vi "Resize Buffer.vi"(8 "error in (no error)":errorcluster, 10 "New Size":i32=-1, 11 "2D U16 DVR Array in":refnum<class "2D U16 DVR Array.lvclass">) -> (0 "error out":errorcluster, 3 "2D U16 DVR Array out":refnum<class "2D U16 DVR Array.lvclass">)   [LabVIEW 2024, in "2D U16 DVR Array.lvclass"]
uses:
  2D U16 DVR Array.lvclass
  2D U16 DVR Array.lvclass/2D U16 DVR Array.ctl
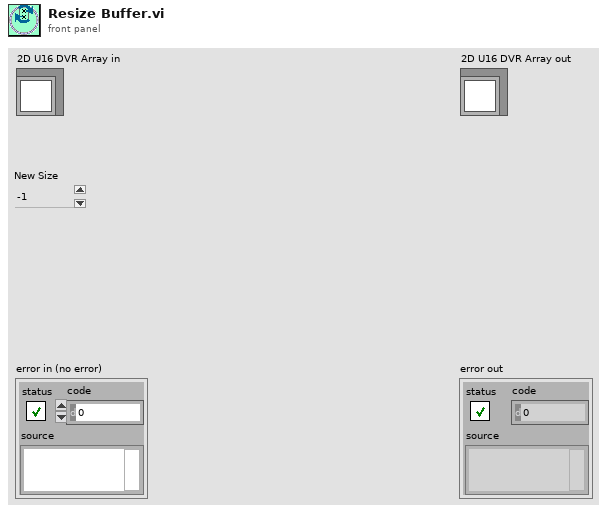
[diagram p1: front panel]
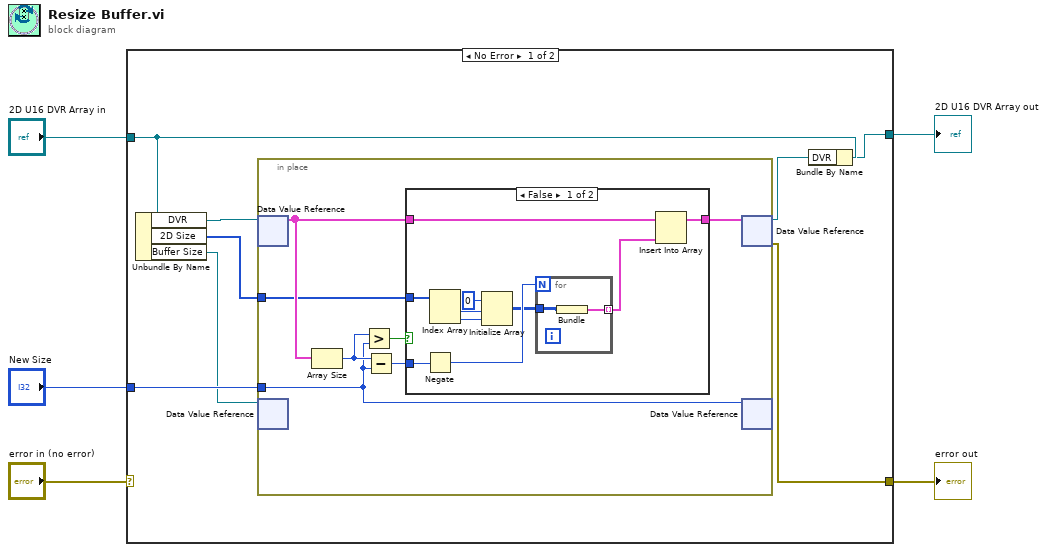
[diagram p0: block diagram]
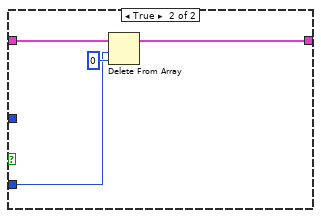
[diagram p2: hidden frame]
diagram:
  n1 = case shown="No Error" "error in (no error)" {
    selector: "error in (no error)" -> [_ w38]
    tunnel: "New Size" -> [w7 _]
    tunnel: [w11 w38] -> w4
    tunnel: "2D U16 DVR Array in" -> [w10 w37]
    tunnel: [w8 w37] -> w1
    frame No Error {
      n2 = Unbundle By Name(w10) -> ("DVR"=w13:refnum<data-value>, "2D Size"=w12:i32[], "Buffer Size"=w6:refnum<data-value>)
      n3 = in-place {
        in-place-border: w7 -> [w14]
        in-place-border: w12 -> [w15]
        n4 = in-place-dvr #1(w13) -> (w19:cluster{u16[][]}[])  [unwired: 1 out]
        n5 = in-place-dvr #2(w6) -> ()  [unwired: 2 out]
        n6 = Array Size(array=w19) -> (size(s)=w17:i32)
        n7 = Greater?(x=w17, y=w14) -> (0:w20:bool)
        n8 = Subtract(x=w17, y=w14) -> (x-y=w18:i32)
        n9 = case shown="False" w20 {
          tunnel: w19 -> [w23 w36]
          tunnel: w18 -> [w30 w34]
          tunnel: [w21 w33] -> w16
          tunnel: w15 -> [w29 _]
          frame False {
            n10 = Negate(x=w30) -> (-x=w25:i32)
            n11 = Index Array(array=w29) -> (element #1=w28:i32, element #2=w27:i32)  [unwired: 2 in]
            n12 = Initialize Array(u16 0 ("element"), w28, w27) -> (w24:u16[][])
            n13 = for {
              N: w25 -> [_]
              tunnel: w24 -> [w32]
              tunnel: [w31] -> w22 mode=indexing
              n14 = Bundle(w32) -> (w31:cluster{u16[][]})  [unwired: 1 in]
            }
            n15 = Insert Into Array(array=w23, new element=w22) -> (w21:cluster{u16[][]}[])  [unwired: 1 in]
          }
          frame True {
            n16 = Delete From Array(array=w36, length=w34, index=0) -> (array with subset deleted=w33:cluster{u16[][]}[])  [unwired: 1 out]
          }
        }
        n17 = in-place-dvr #1(w16) -> (w9:refnum<data-value>, w11:errorcluster)
        n18 = in-place-dvr #2(w14) -> ()  [unwired: 2 out]
      }
      n19 = Bundle By Name(cluster=w10, "DVR"=w9) -> (w8:refnum<class "2D U16 DVR Array.lvclass">)
    }
    frame Error {
    }
  }
  "error out" <- w4
  "2D U16 DVR Array out" <- w1
